vi "String to 2D I64 Array.vi"(6 "Delimiter (,)":string=",", 8 "error in (no error)":errorcluster, 11 "String":string) -> (0 "error out":errorcluster, 3 "2D Array":i64[][](array[numeric]))   [LabVIEW 2016, in "SLL String.lvlib"]
uses:
  SLL String.lvlib
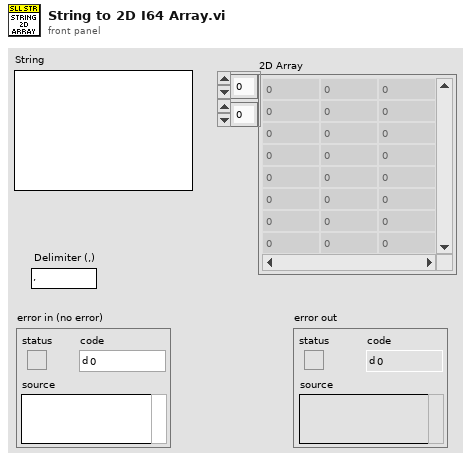
[diagram p1: front panel]
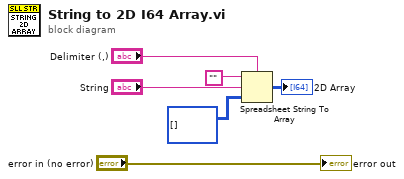
[diagram p0: block diagram]
diagram:
  n1 = Spreadsheet String To Array(delimiter (Tab)="Delimiter (,)", format string="", spreadsheet string="String", array type (2D Dbl)=i64[][] []) -> (array=→"2D Array":i64[][])
  "error out" <- "error in (no error)"
